vi "start_sweep.vi"(8 "error in (no error)":errorcluster, 11 "ImagingModeDL090130Frame in":refnum<class "ImagingModeDL090130Frame.lvclass">=refnum) -> (0 "error out":errorcluster, 3 "ImagingModeDL090130Frame out":refnum<class "ImagingModeDL090130Frame.lvclass">)   [LabVIEW 2010, in "ImagingModeDL090130Frame.lvclass"]
uses:
  ImagingModeDL090130Frame.lvclass
  ImagingModeDL090923Scaffold/ImagingModeDL090923Scaffold/ImagingModeDL090923Scaffold.lvclass
  ImagingModeDL090130Frame.lvclass/ImagingModeDL090130Frame.ctl
  common/xcontrols/XIntensityCompensation/XIntensityCompensation/XIntensityCompensation.xctl
  common/classes/GenericComponent/GenericComponent/class_data.vi
  common/classes/ErrorController/ErrorController/class_data.vi
  common/classes/ErrorController/ErrorController/ErrorController.lvclass
  common/classes/GenericComponent/GenericComponent/GenericComponent.lvclass
  Stage/GenericStage/GenericStage/GenericStage.lvclass
  Stage/GenericStage/GenericStage/trigger_enum.ctl
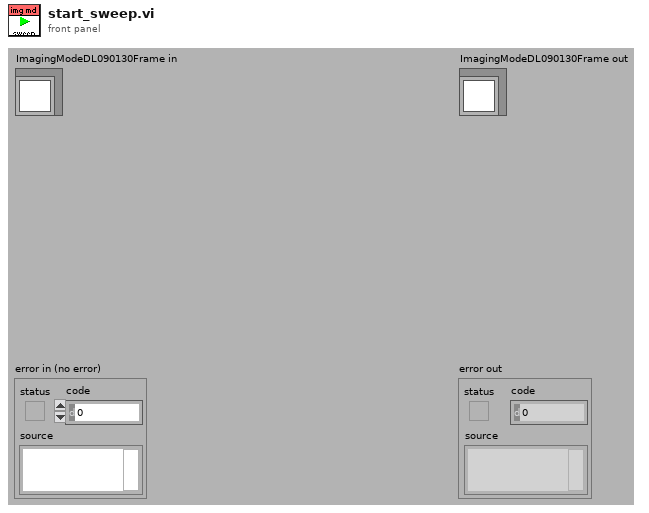
[diagram p1: front panel]
types:
  T1 = typedef "GenericStage.lvclass/trigger_enum.ctl" = enum16{"NULL", "move", "update position", "set origin", "return to origin"}
  T2 = typedef "ImagingModeDL090130Frame.lvclass/translation_mode_enum.ctl" = enum16{"scanHead", "stage"}
  T3 = typedef "ImagingModeDL090130Frame.lvclass/control_refs.ctl" = cluster{"resolution controls":cluster{"x pixels":refnum<vi>, "y pixels":refnum<vi>, "ratio x factor":refnum<vi>, "ratio y factor":refnum<vi>, "Vy min(V)":refnum<vi>, "Vy max(V)":refnum<vi>, "Vz min(V)":refnum<vi>, "Vz max(V)":refnum<vi>}, "speed controls":cluster{"pixel dwell time":refnum<vi>, "line scan time":refnum<vi>, "frame rate":refnum<vi>, "keep constant":refnum<vi>}, "number of frames controls":cluster{"# of frames":refnum<vi>, "duration":refnum<vi>, "# of repetitions":refnum<vi>}, "current value indicators":cluster{"frame #":refnum<vi>, "repetition #":refnum<vi>, "offset":refnum<vi>}, "step controls":cluster{"step size":refnum<vi>, "return to origin?":refnum<vi>, "translation mode":refnum<vi>, "XIntensityCompensation":refnum<vi>}, "defineButton":refnum<vi>, "settings enforced?":refnum<vi>, "settings":refnum<vi>}
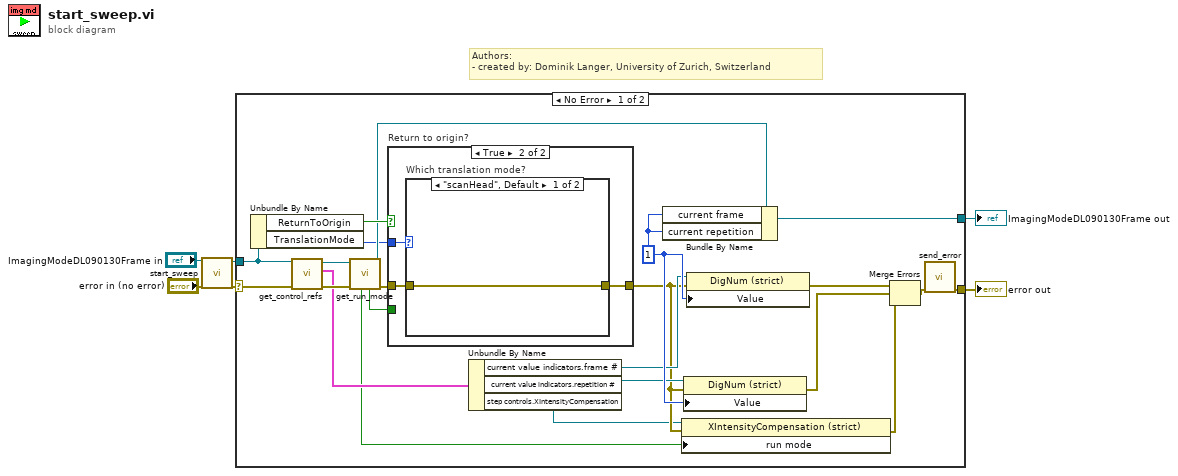
[diagram p0: block diagram]
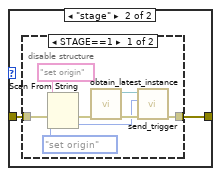
[diagram p3: hidden frame]
diagram:
  # "Authors: \n- created by: Dominik Langer, University of Zurich, Switzerland"
  n1 = call-parent "start_sweep.vi"("error in (no error)"="error in (no error)", "ScanModeDL090923Scaffold in"="ImagingModeDL090130Frame in") -> ("error out"=w3:errorcluster, "ScanModeDL090923Scaffold out"=w1:refnum<class "ImagingModeDL090130Frame.lvclass">)  [unwired: 8 in]
  n2 = case shown="No Error" w3 {
    selector: w3 -> [w25 w46]
    tunnel: [w26 w46] -> w6
    tunnel: [w22 w45] -> w5
    tunnel: w1 -> [w14 w45]
    frame No Error {
      w28 = 1 ("current frame")
      n3 = Unbundle By Name(w14) -> ("ReturnToOrigin"=w27:bool, "TranslationMode"=w7:T2)
      n4 = call-dynamic "get_control_refs.vi"("error in (no error)"=w25, "ImagingModeDL090130Frame in"=w14) -> ("error out"=w24:errorcluster, "control refs"=w10:T3, "ImagingModeDL090130Frame out"=w16:refnum<class "ImagingModeDL090130Frame.lvclass">)  [unwired: 7 in]
      n5 = call "get_run_mode.vi"("error in (no error)"=w24, "GenericPlugin in"=w16) -> ("error out"=w23:errorcluster, "GenericPlugin out"=w15:refnum<class "ImagingModeDL090130Frame.lvclass">, "is NOT free run?"=w11:bool, "is free run?"=w8:bool)  [unwired: 5 in, 1 out]
      n6 = case "Return to origin?" shown="True" w27 {
        tunnel: w23 -> [w29 w32]
        tunnel: [w29 w31] -> w13
        tunnel: w11 -> [_ _]
        tunnel: w7 -> [_ w30]
        frame False {
        }
        frame True {
          n7 = case "Which translation mode?" shown="\"scanHead\", Default" w30 {
            tunnel: w32 -> [w33 w35]
            tunnel: [w33 w34] -> w31
            frame "scanHead", Default {
            }
            frame "stage" {
              n8 = disable-structure shown="STAGE==1" {
                disable-tunnel: w35 -> [w40 w44]
                disable-tunnel: [w42 w44] -> w34
                frame condition #0 {
                  n9 = Scan From String(input string="set origin", error in=w40, default 1=trigger_enum."set origin" ("trigger")) -> (error out=w39:errorcluster, output 1=w37:T1)  [unwired: 2 in, 2 out]
                  n10 = call "obtain_latest_instance.vi"("error in (no error)"=w39) -> ("error out"=w43:errorcluster, "GenericStage out"=w41:refnum<class "GenericStage.lvclass">)  [unwired: 9 in]
                  n11 = call-dynamic "send_trigger.vi"("error in (no error)"=w43, "trigger"=w37, "GenericStage in"=w41) -> ("error out"=w42:errorcluster)  [unwired: 7 in, 1 out]
                }
                frame condition #1 (active) {
                }
              }
            }
          }
        }
      }
      n12 = Unbundle By Name(w10) -> ("current value indicators.frame #"=w21:refnum<vi>, "current value indicators.repetition #"=w20:refnum<vi>, "step controls.XIntensityCompensation"=w9:refnum<vi>)
      n13 = Bundle By Name(cluster=w15, "current frame"=w28, "current repetition"=w28) -> (w22:refnum<class "ImagingModeDL090130Frame.lvclass">)
      n14 = property class="XIntensityCompensation (strict)"(reference=w9, error in=w13, "run mode"=w8) -> (error out=w12:errorcluster)  [unwired: 1 out]
      n15 = property class="DigNum (strict)"(reference=w20, error in=w13, "Value"=w28) -> (error out=w19:errorcluster)  [unwired: 1 out]
      n16 = property class="DigNum (strict)"(reference=w21, error in=w13, "Value"=w28) -> (error out=w18:errorcluster)  [unwired: 1 out]
      n17 = Merge Errors(w18, w19, w12) -> (w17:errorcluster)
      n18 = call "send_error.vi"("error in (no error)"=w17) -> ("error out"=w26:errorcluster)  [unwired: 10 in]
    }
    frame Error {
    }
  }
  "error out" <- w6
  "ImagingModeDL090130Frame out" <- w5
